vi "rhoplusdot_decay.vi"(9 "rho- in":dbl[](array[numeric]), 10 "rho0 in":dbl[](array[numeric]), 11 "rho+ in":dbl[](array[numeric])) -> (3 "rho+ dot out":dbl[](array[numeric]))   [LabVIEW 2018]
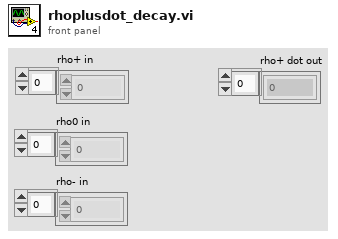
[diagram p1: front panel]
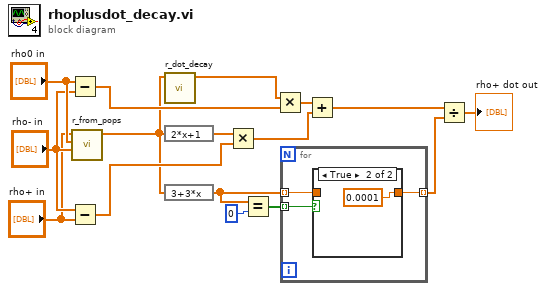
[diagram p0: block diagram]
diagram:
  n1 = Subtract(x="rho0 in", y="rho- in") -> (x-y=w13:dbl[])
  n2 = Subtract(x="rho- in", y="rho+ in") -> (x-y=w16:dbl[])
  n3 = call "r_from_pops.vi"("rho- in"="rho- in", "rho0 in"="rho0 in", "rho+ in"="rho+ in") -> ("r array out"=w3:dbl[])  [unwired: 8 in]
  n4 = call "r_dot_decay.vi"("r array in"=w3) -> ("r dot out"=w2:dbl[])  [unwired: 10 in]
  n5 = expression code="2*x+1"(w3) -> (w5:dbl[])
  n6 = expression code="3+3*x"(w3) -> (w9:dbl[])
  n7 = Multiply(x=w5, y=w16) -> (x*y=w15:dbl[])
  n8 = Equal?(x=w9, y=0) -> (x = y?=w10:bool[])
  n9 = Multiply(x=w2, y=w13) -> (x*y=w6:dbl[])
  n10 = for {
    tunnel: w10 -> [w19] mode=indexing
    tunnel: w9 -> [w18] mode=indexing
    tunnel: [w17] -> w8 mode=indexing
    n11 = case shown="True" w19 {
      tunnel: w18 -> [w20 _]
      tunnel: [w20 0.0001] -> w17
      frame False {
      }
      frame True {
      }
    }
  }
  n12 = Add(x=w6, y=w15) -> (x+y=w7:dbl[])
  n13 = Divide(x=w7, y=w8) -> (x/y=→"rho+ dot out":dbl[])
